vi "DST800全局变量.vi"() -> ()   [LabVIEW 2016, in "DST800.lvlib"]
uses:
  DST800.lvlib
panel:
  out "serial error out":errorcluster
  out "depth":cluster{"时间标识":timestamp, "深度":dbl}
  in  "DST800 串口":refnum<visa-resource-name>="COM9"
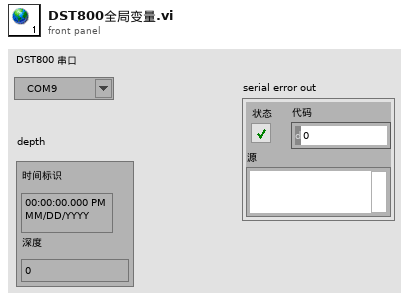
[diagram p1: front panel]
diagram:
